vi "BtoI.vi"(11 "Field":dbl) -> (3 "Current":dbl)   [LabVIEW 2013]
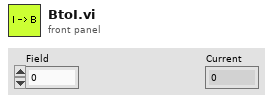
[diagram p1: front panel]
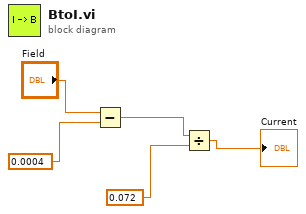
[diagram p0: block diagram]
diagram:
  n1 = Subtract(x="Field", y=0.0004) -> (x-y=w3:dbl)
  n2 = Divide(x=w3, y=0.072) -> (x/y=→"Current":dbl)
